vi "get available devices.vi"(8 "error in (no error)":errorcluster, 11 "BMC in":refnum<class "BMC.lvclass">) -> (0 "error out":errorcluster {"code" format="%.0x"}, 3 "BMC out":refnum<class "BMC.lvclass">)   [LabVIEW 2012, in "BMC.lvclass"]
uses:
  BMC.lvclass
  BMC.lvclass/BMC.ctl
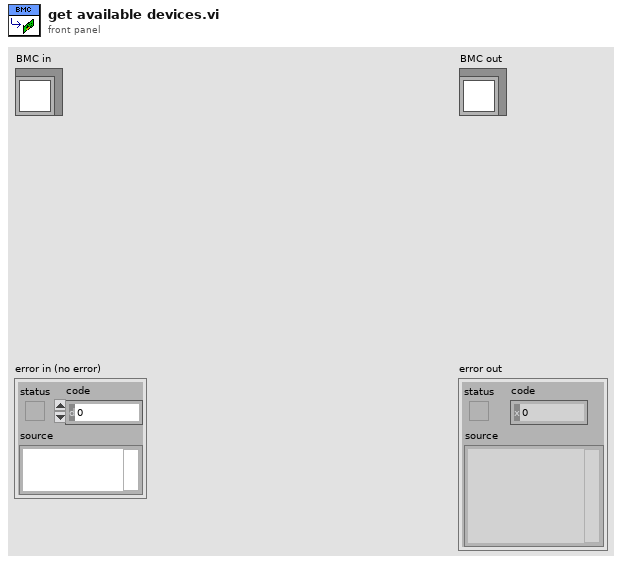
[diagram p1: front panel]
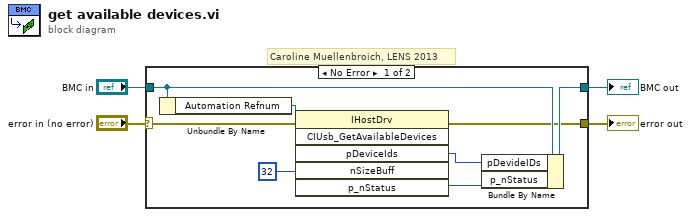
[diagram p0: block diagram]
diagram:
  # "Caroline Muellenbroich, LENS 2013"
  n1 = case shown="No Error" "error in (no error)" {
    selector: "error in (no error)" -> [w12 w14]
    tunnel: [w7 w14] -> w3
    tunnel: [w10 w13] -> w1
    tunnel: "BMC in" -> [w9 w13]
    frame No Error {
      n2 = Unbundle By Name(w9) -> ("Automation Refnum"=w8:refnum<k7>)
      n3 = invoke class="IHostDrv" method="CIUsb_GetAvailableDevices"(reference=w8, error in=w12, "nSizeBuff"=32 ("dimension size")) -> (error out=w7:errorcluster, "pDeviceIds"=w6:i32, "p_nStatus"=w5:i32)  [unwired: 3 in, 3 out]
      n4 = Bundle By Name(cluster=w9, "pDevideIDs"=w6, "p_nStatus"=w5) -> (w10:refnum<class "BMC.lvclass">)
    }
    frame Error {
    }
  }
  "error out" <- w3
  "BMC out" <- w1
